vi "Time.Date String to Time Stamp.vi"(7 "Format":string="%<%m/%d/%Y>T", 8 "Error In":errorcluster, 11 "Date Str(mm/dd/yyyy)":string) -> (0 "Error Out":errorcluster, 1 "Days Away":dbl, 2 "Past":bool, 3 "Time Stamp":timestamp)   [LabVIEW 2024, in "EQMF.lvlib" / "Time Utils.lvlib"]
doc: "This VI converts a date string to a time stamp. The time stamp will be set to noon of the date entered.\n\nThe default format is \"%<%m/%d/%Y>T\" (Month/Day/4 digit Year). If the input string format is different use the 'Format' input to indicate the appropriate format:\n %Y = 4 digit year\n %y = 2 digit year\n %m = month\n %d = day\n\nEXAMPLE: for Year-Month-Day use format: \"%<%Y-%m-%d>T\""
uses:
  Time Utils.lvlib
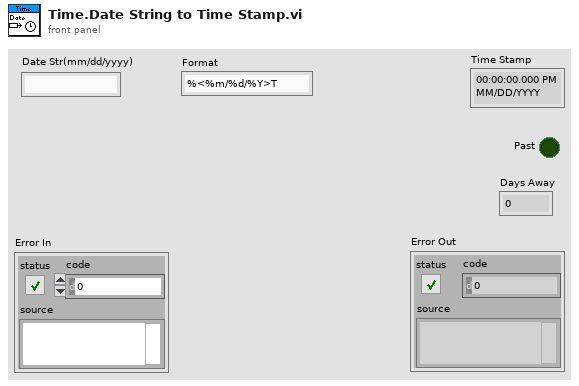
[diagram p1: front panel]
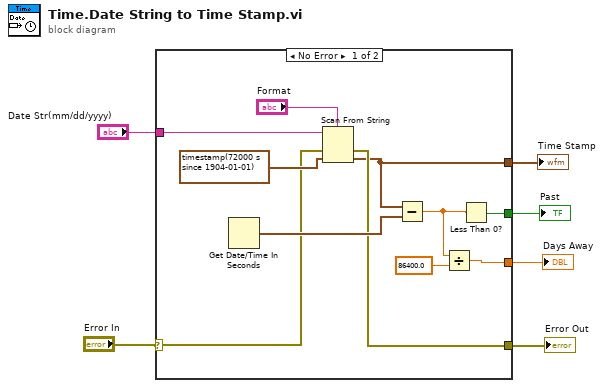
[diagram p0: block diagram]
diagram:
  n1 = case shown="No Error" "Error In" {
    selector: "Error In" -> [w8 w18]
    tunnel: "Date Str(mm/dd/yyyy)" -> [w15 _]
    tunnel: [w7 _] -> w5
    tunnel: [w12 _] -> w4
    tunnel: [w10 _] -> w3
    tunnel: [w9 w18] -> w2
    frame No Error {
      n2 = Get Date/Time In Seconds() -> (seconds since 1Jan1904=w14:timestamp)
      n3 = Scan From String(format string="Format", input string=w15, error in=w8, default 1=timestamp(72000 s since 1904-01-01)) -> (error out=w9:errorcluster, output 1=w7:timestamp)  [unwired: 1 in, 2 out]
      n4 = Subtract(x=w7, y=w14) -> (x-y=w11:dbl)
      n5 = Divide(x=w11, y=86400.0) -> (x/y=w12:dbl)
      n6 = Less Than 0?(x=w11) -> (x < 0?=w10:bool)
    }
    frame Error {
    }
  }
  "Time Stamp" <- w5
  "Past" <- w3
  "Days Away" <- w4
  "Error Out" <- w2
